vi "Ingest Data.vi"(8 "error in":errorcluster, 10 "NewData":refnum<class "CRDS Data.lvclass">, 11 "OldData":refnum<class "CRDS Data.lvclass">) -> (0 "error out":errorcluster, 3 "CRDS Data out":refnum<class "CRDS Data.lvclass">)   [LabVIEW 2014, in "CRDS Data.lvclass"]
uses:
  CRDS Data.lvclass
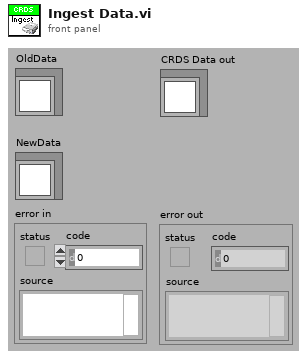
[diagram p1: front panel]
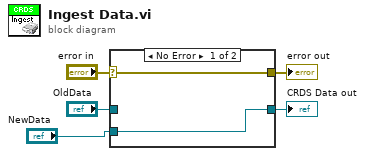
[diagram p0: block diagram]
diagram:
  n1 = case shown="No Error" "error in" {
    selector: "error in" -> [w7 w9]
    tunnel: [w7 w9] -> w4
    tunnel: [w6 w8] -> w2
    tunnel: "OldData" -> [_ w8]
    tunnel: "NewData" -> [w6 _]
    frame No Error {
    }
    frame Error {
    }
  }
  "error out" <- w4
  "CRDS Data out" <- w2
